vi "Query with 2D 64bit Integer Result.vi"(8 "error in (no error)":errorcluster, 10 "Query string":string, 11 "sqlite3 in":refnum<class "sqlite3.lvclass">) -> (0 "error out":errorcluster, 2 "Result":i64[][](array[numeric]), 3 "sqlite3 out":refnum<class "sqlite3.lvclass">)   [LabVIEW 2020, in "sqlite3.lvlib" / "sqlite3.lvclass"]
uses:
  sqlite3.lvclass
  sqlite3.lvclass/sqlite3.ctl
  0c059362-b9b9-4866-9b37-044a88fc3634.vi
  sqlite/VIs/open v2.vi
  sqlite/VIs/close v2.vi
  sqlite/VIs/prepare v2.vi
  sqlite/VIs/step.vi
  sqlite/VIs/column count.vi
  db layer/compound/Resolve Result Type.vi
  0c059362-b9b9-4866-9b37-044a88fc3634.vi/7bc19fd7-2686-4951-aa35-a0d62870a61f.vi
  0c059362-b9b9-4866-9b37-044a88fc3634.vi/0c990a8c-7110-4797-b890-0104de729f69.vi
  sqlite/VIs/finalize.vi
  sqlite/subvi/Error Converter (ErrCode or Status).vi
  sqlite/VIs/column type.vi
  sqlite/VIs/column int64.vi
  0c059362-b9b9-4866-9b37-044a88fc3634.vi/7bc19fd7-2686-4951-aa35-a0d62870a61f.vi/c3a74749-1ef8-497f-bac9-7930eb10c389.vi
  sqlite/VIs/errstr.vi
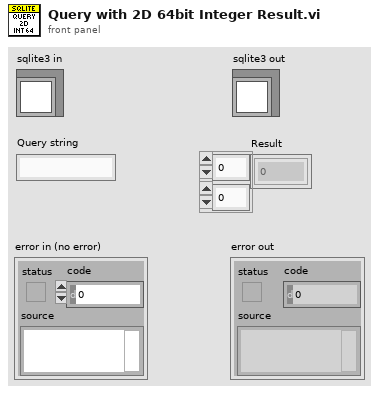
[diagram p1: front panel]
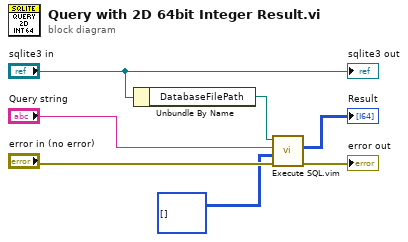
[diagram p0: block diagram]
diagram:
  n1 = Unbundle By Name("sqlite3 in") -> ("DatabaseFilePath"=w7:path)
  n2 = call "Execute SQL.vim"("error in (no error)"="error in (no error)", "desired return type(none)"=i64[][] [] ("Result 2"), "sql (string)"="Query string", "database in"=w7) -> ("error out"=→"error out":errorcluster, "Query Result"=→"Result":i64[][])  [unwired: 6 in]
  "sqlite3 out" <- "sqlite3 in"
